vi "Spartan HTTP Destroy Session.vi"(8 "error in (no error)":errorcluster, 11 "object":T1 {"object data"."time" format="%0.2f"}) -> (0 "error out":errorcluster)   [LabVIEW 2011]
doc: "Function that cleans up when an object is destroyed.\nIt may close a file or connection, or may need to trigger an occurrence."
uses:
  Spartan HTTP Session.ctl
  ITK EXT/http/http_obj.llb/HTTP Session Data.ctl
  ITK EXT/utils/keyedarr.llb/Keyed Array.ctl
  ITK EXT/http/cookie.llb/Cookie.ctl
panel:
  out "TCP CLOSE error out":errorcluster
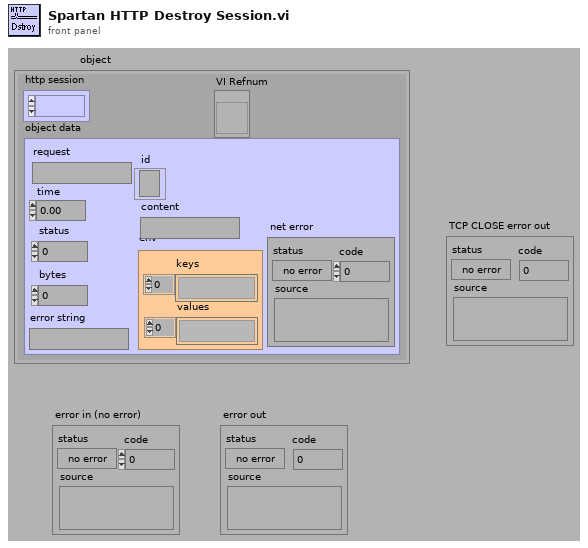
[diagram p1: front panel]
types:
  T1 = typedef "Spartan HTTP Session.ctl" = cluster{"http session":refnum<k1>, "object data":T2, "VI Refnum":refnum<vi>}
  T2 = typedef "HTTP Session Data.ctl" = cluster{"request":string, "time":dbl, "status":i32, "error string":string, "bytes":i32, "env":T3, "content":string, "id":refnum<k5>, "net error":errorcluster}
  T3 = typedef "Keyed Array.ctl" = cluster{"keys":string[], "values":string[]}
  T4 = typedef "Cookie.ctl" = cluster{"cookie id":string, "address":string}
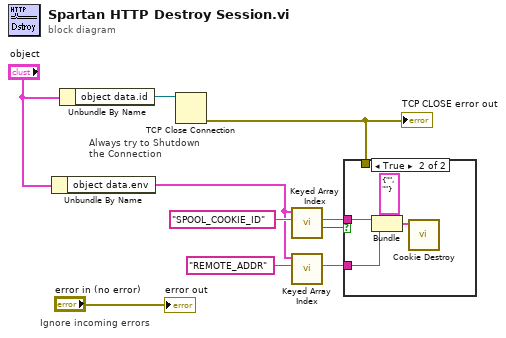
[diagram p0: block diagram]
diagram:
  # "Always try to Shutdown\nthe Connection"
  # "Ignore incoming errors"
  n1 = Unbundle By Name("object") -> ("object data.env"=w5:T3)
  n2 = Unbundle By Name("object") -> ("object data.id"=w10:refnum<k5>)
  n3 = TCP Close Connection(connection ID=w10) -> (error out=w2:errorcluster)  [unwired: 1 in, 2 out]
  "TCP CLOSE error out" <- w2
  n4 = call "Keyed Array Index.vi"("key"="SPOOL_COOKIE_ID", "array in"=w5) -> ("valid key"=w8:bool, "value"=w7:string)  [unwired: 2 in, 2 out]
  n5 = call "Keyed Array Index.vi"("key"="REMOTE_ADDR", "array in"=w5) -> ("value"=w4:string)  [unwired: 2 in, 3 out]
  n6 = case shown="True" w8 {
    tunnel: w7 -> [_ w14]
    tunnel: w4 -> [_ w13]
    tunnel: w2 -> [_ _]
    frame False {
    }
    frame True {
      n7 = Bundle(cluster=T4 {"cookie id"="", "address"=""} ("cookie"), "cookie id"=w14, "address"=w13) -> (w12:T4)
      n8 = call "Cookie Destroy.vi"("cookie"=w12) -> ()  [unwired: 1 in, 10 out]
    }
  }
  "error out" <- "error in (no error)"
